vi "ParseTxResult.vi"(8 "error in (no error)":errorcluster, 11 "Results":string[](array[string])=["1,-15.852258,-4.171936,-16.616194\n", "1,-32.7547,-33.0151,-32.7485\n", "-3.528785,-4.156985,0.733084,0.368447,1,0.021492,0.825732,-38.226673,0.000000\n", "1,7.960808,5299532163.742691,0.000000\n"]) -> (0 "error out":errorcluster, 1 "MASK":dbl, 2 "FreqError":dbl, 3 "EVM":dbl, 5 "TxPower":dbl)   [LabVIEW 2014]
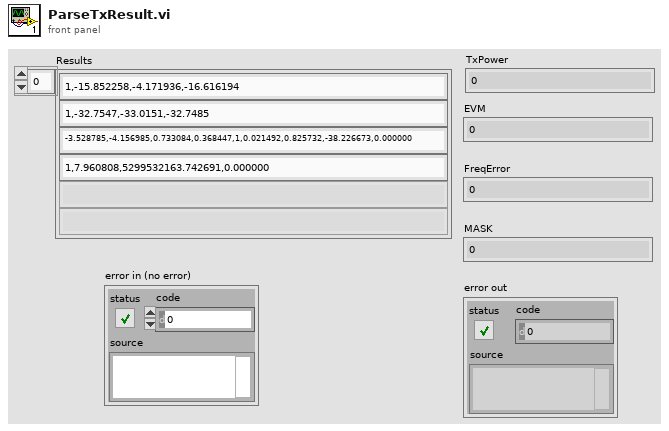
[diagram p1: front panel]
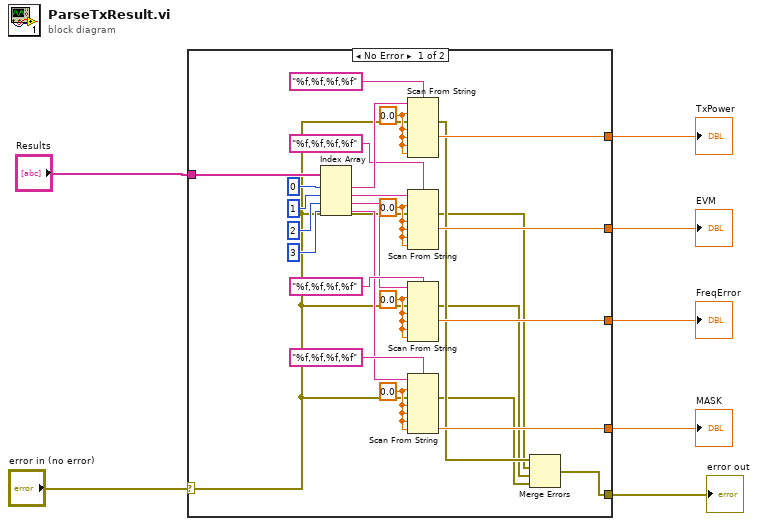
[diagram p0: block diagram]
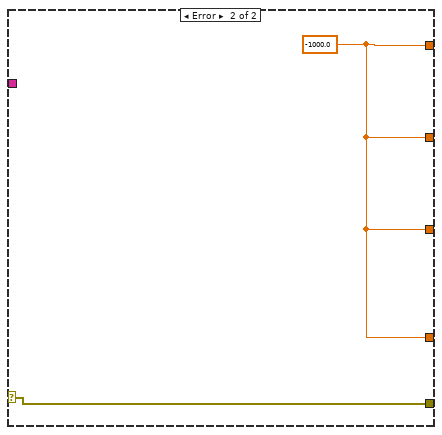
[diagram p2: hidden frame]
diagram:
  n1 = case shown="No Error" "error in (no error)" {
    selector: "error in (no error)" -> [w13 w35]
    tunnel: "Results" -> [w34 _]
    tunnel: [w26 w36] -> w6
    tunnel: [w25 w36] -> w5
    tunnel: [w20 w36] -> w4
    tunnel: [w16 w36] -> w3
    tunnel: [w12 w35] -> w1
    frame No Error {
      w19 = 0.0 ("initial scan location")
      w21 = 0.0 ("initial scan location")
      w24 = 0.0 ("initial scan location")
      w27 = 0.0 ("initial scan location")
      n2 = Index Array(array=w34, index #1=0 ("index"), index #2=1 ("index"), index #3=2 ("index"), index #4=3 ("index")) -> (element #1=w29:string, element #2=w17:string, element #3=w15:string, element #4=w14:string)
      n3 = Scan From String(format string="%f,%f,%f,%f", input string=w29, initial scan location=w27, error in=w13, default 1=w27, default 2=w27, default 3=w27, default 4=w27) -> (error out=w11:errorcluster, output 2=w26:dbl)  [unwired: 3 in, 2 out]
      n4 = Scan From String(format string="%f,%f,%f,%f", input string=w17, initial scan location=w24, error in=w13, default 1=w24, default 2=w24, default 3=w24, default 4=w24) -> (error out=w10:errorcluster, output 2=w25:dbl)  [unwired: 3 in, 2 out]
      n5 = Scan From String(format string="%f,%f,%f,%f", input string=w15, initial scan location=w21, error in=w13, default 1=w21, default 2=w21, default 3=w21, default 4=w21) -> (error out=w9:errorcluster, output 2=w20:dbl)  [unwired: 3 in, 2 out]
      n6 = Scan From String(format string="%f,%f,%f,%f", input string=w14, initial scan location=w19, error in=w13, default 1=w19, default 2=w19, default 3=w19, default 4=w19) -> (error out=w8:errorcluster, output 4=w16:dbl)  [unwired: 3 in, 2 out]
      n7 = Merge Errors(w11, w10, w9, w8) -> (w12:errorcluster)
    }
    frame Error {
      w36 = -1000.0 ("initial scan location")
    }
  }
  "TxPower" <- w6
  "EVM" <- w5
  "FreqError" <- w4
  "MASK" <- w3
  "error out" <- w1
